vi "例7.5利用XY图显示多条曲线.vi"() -> ()   [LabVIEW 2017]
panel:
  out "4（X和Y数组）多条曲线":cluster{i32[], dbl[]}[](graph)
  out "3（X和Y数组）单条曲线":cluster{i32[], dbl[]}(graph)
  out "2（Array of Pts）多条曲线":cluster{cluster{i32, dbl}[]}[](graph)
  out "1（Array of Pts）单条曲线":cluster{i32, dbl}[](graph)
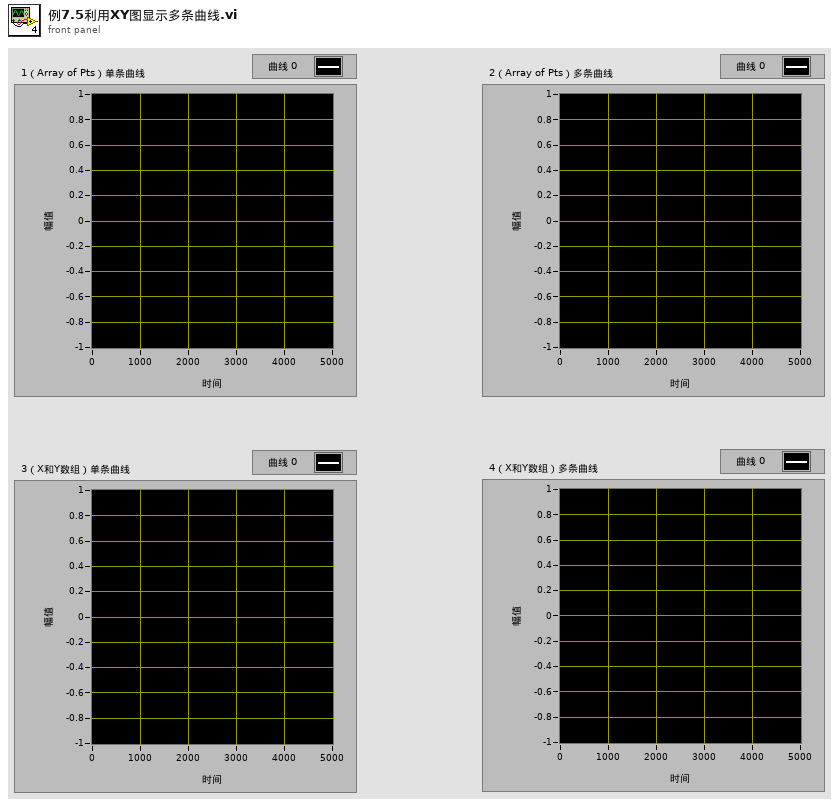
[diagram p1: front panel]
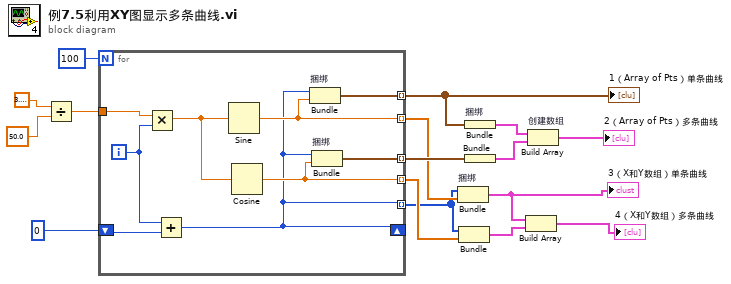
[diagram p0: block diagram]
diagram:
  n1 = Divide(x=3.141592653589793, y=50.0) -> (x/y=w13:dbl)
  n2 = for {
    N: 100 -> [_]
    tunnel: w13 -> [w25]
    tunnel: [w21] -> w7 mode=indexing
    tunnel: [w20] -> w6 mode=indexing
    shift-right: [w17] -> _
    shift-left: 0 -> [w23]
    tunnel: [w19] -> w1 mode=indexing
    tunnel: [w18] -> w11 mode=indexing
    tunnel: [w17] -> w4 mode=indexing
    i -> [w22]
    n3 = Multiply(x=w25, y=w22) -> (x*y=w24:dbl)
    n4 = Add(x=w22, y=w23) -> (x+y=w17:i32)
    n5 = Sine(x=w24) -> (sin(x)=w21:dbl)
    n6 = Cosine(x=w24) -> (cos(x)=w20:dbl)
    n7 = Bundle "捆绑"(w17, w21) -> (w19:cluster{i32, dbl})  [unwired: 1 in]
    n8 = Bundle "捆绑"(w17, w20) -> (w18:cluster{i32, dbl})  [unwired: 1 in]
  }
  "1（Array of Pts）单条曲线" <- w1
  n9 = Bundle "捆绑"(w4, w7) -> (w3:cluster{i32[], dbl[]})  [unwired: 1 in]
  "3（X和Y数组）单条曲线" <- w3
  n10 = Bundle(w4, w6) -> (w5:cluster{i32[], dbl[]})  [unwired: 1 in]
  n11 = Bundle "捆绑"(w1) -> (w10:cluster{cluster{i32, dbl}[]})  [unwired: 1 in]
  n12 = Bundle(w11) -> (w9:cluster{cluster{i32, dbl}[]})  [unwired: 1 in]
  n13 = Build Array(w3, w5) -> (→"4（X和Y数组）多条曲线":cluster{i32[], dbl[]}[])
  n14 = Build Array "创建数组"(w10, w9) -> (→"2（Array of Pts）多条曲线":cluster{cluster{i32, dbl}[]}[])
